vi "Read RFx.vi"(8 "error in (no error)":errorcluster, 11 "WS5100 in":refnum<class "WS5100.lvclass">) -> (0 "error out":errorcluster, 2 "RFx":bool[](array[boolean])=[TRUE, TRUE, TRUE, TRUE], 3 "WS5100 out":refnum<class "WS5100.lvclass">)   [LabVIEW 2020, in "WS5100.lvclass"]
uses:
  WS5100.lvclass
  WS5100.lvclass/WS5100.ctl
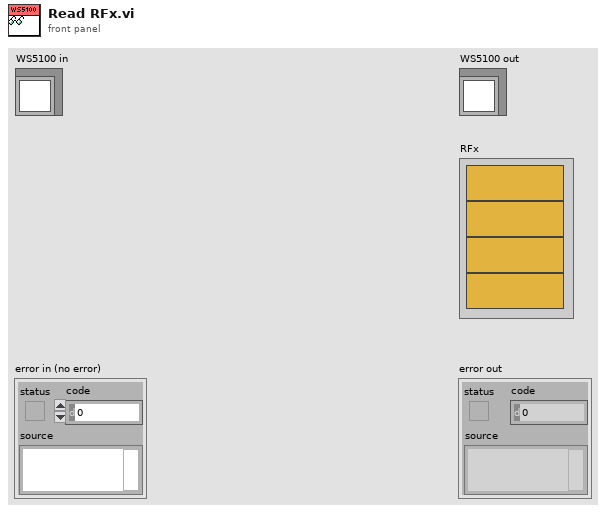
[diagram p1: front panel]
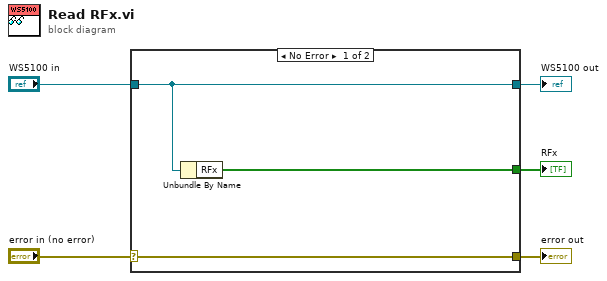
[diagram p0: block diagram]
diagram:
  n1 = case shown="No Error" "error in (no error)" {
    selector: "error in (no error)" -> [w8 w9]
    tunnel: [w8 w9] -> w4
    tunnel: [w7 w10] -> w2
    tunnel: "WS5100 in" -> [w7 w10]
    tunnel: [w6 _] -> w1
    frame No Error {
      n2 = Unbundle By Name(w7) -> ("RFx"=w6:bool[])
    }
    frame Error {
    }
  }
  "error out" <- w4
  "WS5100 out" <- w2
  "RFx" <- w1
